vi "write.vi"   [LabVIEW 2015, in "lv-graph-global.lvlib"]
uses:
  lv-graph-global.lvlib
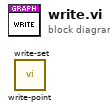
[diagram p0: block diagram]
diagram:
  n1 = call "write-point.vi"() -> ()  [unwired: 10 in, 2 out]
  n2 = call "write-set.vi"() -> ()  [unwired: 11 in, 1 out]
